vi "Add Alias.vi"(8 "error in":errorcluster, 9 "endpoint":T1, 10 "alias":string, 11 "endpoint aliases in":T2 format="%.0x") -> (0 "error out":errorcluster, 3 "endpoint aliases out":T2 format="%.0x")   [LabVIEW 2020, in "Routing and Faulting Scripting.lvlib"]
doc: "Creates an alias for the specified endpoint. This alias is displayed in the Routing and Faulting custom device."
uses:
  Routing and Faulting Scripting.lvlib
  <vilib>/NI VeriStand/Custom Device API/Custom Device Item Ref.ctl
  Shared/Alias Endpoint.ctl
  <vilib>/NI VeriStand/Custom Device API/Get Item Property (String).vi
  <vilib>/NI VeriStand/Custom Device API/Custom Device API.lvlib
  Shared/Routing and Faulting Shared.lvlib
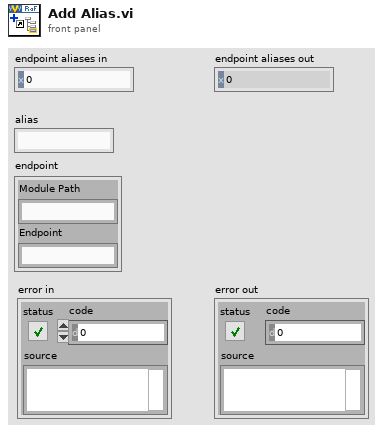
[diagram p1: front panel]
types:
  T1 = typedef "Routing and Faulting Shared.lvlib/Alias Endpoint.ctl" = cluster{"Module Path":string, "Endpoint":string}
  T2 = typedef "Custom Device API.lvlib/Custom Device Item Ref.ctl" = u64
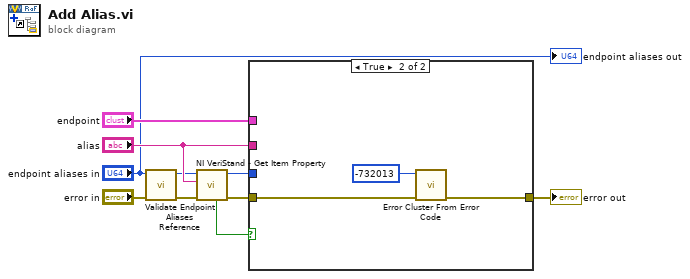
[diagram p0: block diagram]
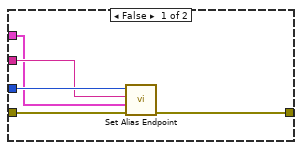
[diagram p2: hidden frame]
diagram:
  n1 = call "Validate Endpoint Aliases Reference.vi"("error in"="error in", "endpoint aliases in"="endpoint aliases in") -> ("error out"=w3:errorcluster, "endpoint aliases out"=w4:T2)  [unwired: 8 in]
  n2 = call-poly <vilib>:"NI VeriStand - Get Item Property.vi"("error in (no error)"=w3, "Property Name"="alias", "Item Ref in"=w4) -> ("error out"=w9:errorcluster, "Item Ref out"=w6:T2, "Found?"=w7:bool)  [unwired: 5 in, 1 out]
  n3 = case shown="True" w7 {
    tunnel: [w14 w16] -> w10
    tunnel: w9 -> [w15 w17]
    tunnel: w6 -> [w13 _]
    tunnel: "alias" -> [w12 _]
    tunnel: "endpoint" -> [w11 _]
    frame False {
      n4 = call "Set Alias Endpoint.vi"("error in"=w15, "new endpoint"=w11, "alias"=w12, "endpoint aliases in"=w13) -> ("error out"=w14:errorcluster)  [unwired: 6 in, 1 out]
    }
    frame True {
      n5 = call <vilib>:"Error Cluster From Error Code.vi"("error in (no error)"=w17, "error code (0)"=-732013) -> ("error out"=w16:errorcluster)  [unwired: 7 in]
    }
  }
  "error out" <- w10
  "endpoint aliases out" <- "endpoint aliases in"
